vi "GetUsrStsBuf.vi"(8 "错误输入（无错误）":errorcluster, 10 "簇":T1, 11 "板卡序号":u8) -> (0 "错误输出":errorcluster, 3 "ppUsrStsBuf":T1)   [LabVIEW 2014]
uses:
  <vilib>/Utility/importsl/GetValueByPointer/datatype.ctl
  <vilib>/Utility/importsl/GetValueByPointer/GetValueByPointer.xnode
  X86Dll/ZXUTConfigMgr.dll
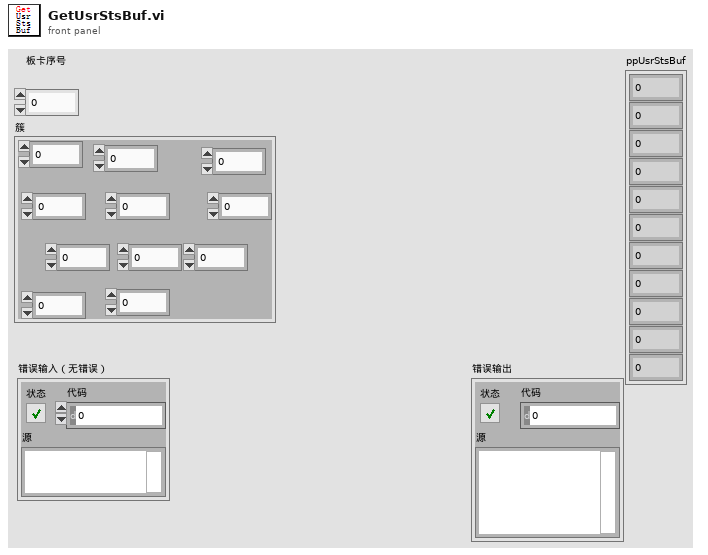
[diagram p1: front panel]
types:
  T1 = cluster{u32, u32, u32, u16, u16, u32, dbl, dbl, dbl, u32, u32}
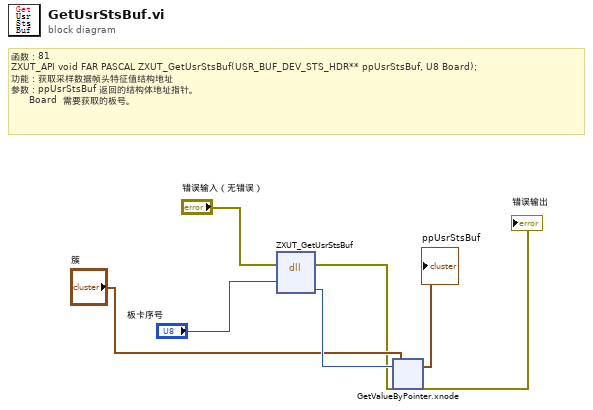
[diagram p0: block diagram]
diagram:
  # "函数：81\nZXUT_API void\tFAR PASCAL ZXUT_GetUsrStsBuf(USR_BUF_DEV_STS_HDR** ppUsrStsBuf, U8 Board);\n功能：获取采样数据帧头特征值结构地址\n参数：ppUsrStsBuf 返回的结构体地址指针。\n      Board  需要获取的板号。"
  n1 = dll-call lib="D:/Software/Utrasonic on-line monitoring/X86Dll/ZXUTConfigMgr.dll" fn="ZXUT_GetUsrStsBuf"(error in="错误输入（无错误）", "Board"="板卡序号") -> (error out=w2:errorcluster, "ppUsrStsBuf"=w5:u64)  [unwired: 5 in, 1 out]
  n2 = xnode "GetValueByPointer.xnode"("Pointer"=w5, "InputType"="簇", "ErrorIn"=w2) -> ("Output"=→"ppUsrStsBuf":T1, "ErrorOut"=→"错误输出":errorcluster)  [unwired: 1 in]
